vi "RTS Find Filename Increment Number.vi"(11 "Input name in":string) -> (1 "After Find":string, 2 "Before Find":string, 3 "Full Input Name":string, 5 "No Match":bool)   [LabVIEW 2016]
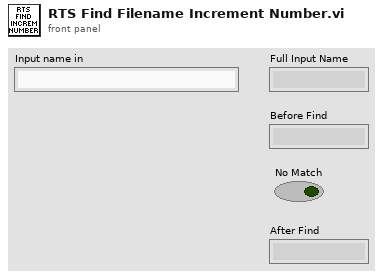
[diagram p1: front panel]
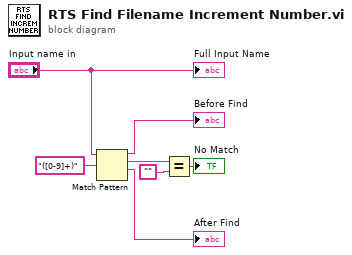
[diagram p0: block diagram]
diagram:
  n1 = Match Pattern(string="Input name in", regular expression="([0-9]+)") -> (before substring=→"Before Find":string, match substring=w3:string, after substring=→"After Find":string)  [unwired: 1 in, 1 out]
  n2 = Equal?(x=w3, y="") -> (x = y?=→"No Match":bool)
  "Full Input Name" <- "Input name in"
